vi "Init Sim Servo Motor.vi"(8 "error in (no error)":errorcluster, 10 "device ID":T1, 11 "NI_Robotics_Starter Kit Host_Sim in":refnum<class "NI_Robotics_Starter Kit Host_Sim.lvclass">) -> (0 "error out":errorcluster, 3 "NI_Robotics_Starter Kit Host_Sim out":refnum<class "NI_Robotics_Starter Kit Host_Sim.lvclass">)   [LabVIEW 2017, in "NI_Robotics_Starter Kit Host_Sim.lvclass"]
uses:
  <vilib>/robotics/Starter Kit/Sim Host Interface/NI_Robotics_Starter Kit Host_Sim.lvclass
  <vilib>/robotics/Simulator/Engine/ctl/DeviceID.ctl
  <vilib>/robotics/Simulator/NI_Robotics_Simulator.lvlib
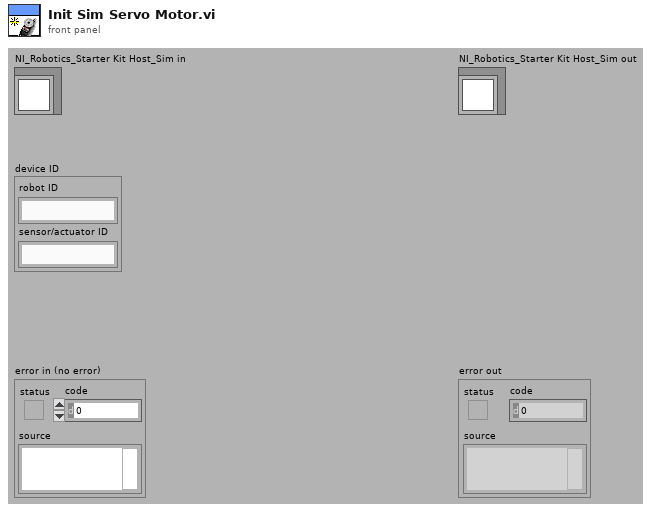
[diagram p1: front panel]
types:
  T1 = typedef "NI_Robotics_Simulator.lvlib/DeviceID.ctl" = cluster{"robot ID":string, "sensor/actuator ID":string}
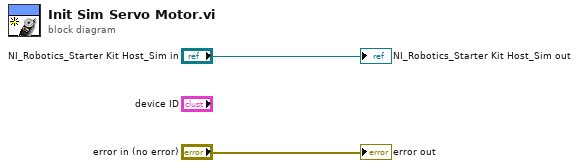
[diagram p0: block diagram]
diagram:
  "error out" <- "error in (no error)"
  "NI_Robotics_Starter Kit Host_Sim out" <- "NI_Robotics_Starter Kit Host_Sim in"
